vi "preparePubDataSVs.vi"(8 "error in (no error)":errorcluster, 11 "Model in":refnum<class "Model.lvclass">) -> (0 "error out":errorcluster, 3 "Model out":refnum<class "Model.lvclass">)   [LabVIEW 2015, in "Model.lvclass"]
doc: "Opens references to the PubDataSVs.\nDetermines the URLs from the configuration and the array of PubDataSVs.\nUpdate the array of PubDataSVs for each component."
uses:
  Model.lvclass
  ComponentTemplateCore/ComponentModel/ComponentModel/Typedefs/CommunicationConfig.ctl
  Typedefs/PubDataSV.ctl
  ComponentTemplateCore/ComponentModel/ComponentModel/Typedefs/SVProcessConfig.ctl
  Model.lvclass/Model.ctl
  Target/Target/Target.lvclass
  Typedefs/EXATypedefs.lvlib
  <vilib>/Utility/VariantDataType/VariantType.lvlib
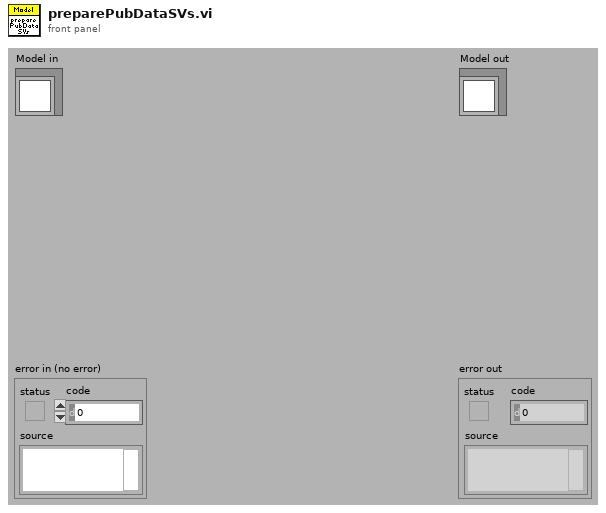
[diagram p1: front panel]
types:
  T1 = typedef "SVProcessConfig.ctl" = cluster{"subDataProcessPrototype":string, "pubDataProcessPrototype":string, "commandProcessPrototype":string, "commandSVName":string}
  T2 = typedef "EXATypedefs.lvlib/PubDataSV.ctl" = enum16{"DetailedState", "ErrorCode", "Heartbeat", "LoopTime_ms", "LoopTimeOutOfRange", "SummaryState", "Timestamp"}
  T3 = typedef "CommunicationConfig.ctl" = cluster{"hostComputerAddress":string, "ComponentAcronym":string, "InstanceIdentifier":i32}
  T4 = cluster{"Read Access":enum8{"Allowed", "Required", "None"}, "Write Access":enum8{"Allowed", "Required", "None"}}
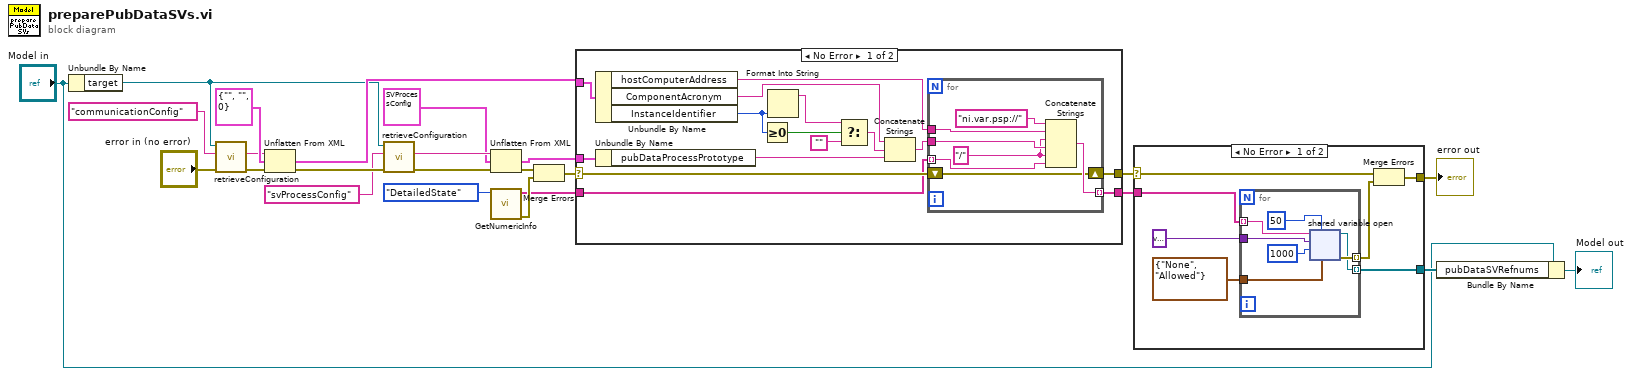
[diagram p0: block diagram]
diagram:
  n1 = Unbundle By Name("Model in") -> ("target"=w1:refnum<class "Target.lvclass">)
  n2 = call-dynamic "retrieveConfiguration.vi"("error in (no error)"="error in (no error)", "dataName"="communicationConfig", "Target in"=w1) -> ("error out"=w15:errorcluster, "dataValueFromFile"=w17:string)  [unwired: 6 in, 1 out]
  n3 = Unflatten From XML(xml string=w17, type=T3 {"hostComputerAddress"="", "ComponentAcronym"="", "InstanceIdentifier"=0} ("sharedVariableLibrariesConfig"), error in (no error)=w15) -> (value=w7:T3, error out=w6:errorcluster)
  n4 = call-dynamic "retrieveConfiguration.vi"("error in (no error)"=w6, "dataName"="svProcessConfig", "Target in"=w1) -> ("error out"=w5:errorcluster, "dataValueFromFile"=w9:string)  [unwired: 6 in, 1 out]
  n5 = Unflatten From XML(xml string=w9, type=T1 {"subDataProcessPrototype"="SubDataSV", "pubDataProcessPrototype"="PubDataSV", "commandProcessPrototype"="CommandSV", "commandSVName"="Command"} ("svProcessConfig"), error in (no error)=w5) -> (value=w2:T1, error out=w4:errorcluster)
  n6 = call <vilib>:"GetNumericInfo.vi"("Variant"=PubDataSV."DetailedState" ("PubDataSV")) -> ("error out"=w13:errorcluster, "EnumNames"=w11:string[])  [unwired: 7 in, 2 out]
  n7 = Merge Errors(w4, w13) -> (w12:errorcluster)
  n8 = case shown="No Error" w12 {
    selector: w12 -> [w34 w47]
    tunnel: [w39 _] -> w21
    tunnel: w7 -> [w37 _]
    tunnel: [w33 w47] -> w22
    tunnel: w11 -> [w27 _]
    tunnel: w2 -> [w26 _]
    frame No Error {
      n9 = Unbundle By Name(w37) -> ("hostComputerAddress"=w36:string, "ComponentAcronym"=w38:string, "InstanceIdentifier"=w32:i32)
      n10 = Unbundle By Name(w26) -> ("pubDataProcessPrototype"=w25:string)
      n11 = Greater Or Equal To 0?(x=w32) -> (x >= 0?=w31:bool)
      n12 = Format Into String(w32) -> (resulting string=w30:string)  [unwired: 3 in, 1 out]
      n13 = Select(t=w30, s=w31, f="") -> (s? t:f=w28:string)
      n14 = Concatenate Strings(w38, w28, w25) -> (w35:string)
      n15 = for {
        tunnel: w36 -> [w45]
        tunnel: w35 -> [w44]
        tunnel: [w42] -> w39 mode=indexing
        shift-right: [w40] -> w33
        shift-left: w34 -> [w40]
        tunnel: w27 -> [w41] mode=indexing
        w43 = "/" ("string")
        n16 = Concatenate Strings("ni.var.psp://" ("string"), w45, w43, w44, w43, w41) -> (w42:string)
      }
    }
    frame Error {
    }
  }
  n17 = case shown="No Error" w22 {
    selector: w22 -> [w52 w62]
    tunnel: w21 -> [w53 _]
    tunnel: [w49 w62] -> w20
    tunnel: [w48 _] -> w19
    frame No Error {
      n18 = for {
        tunnel: T4 {"Read Access"=enum."None", "Write Access"=enum."Allowed"} ("access") -> [w61]
        tunnel: w53 -> [w60] mode=indexing
        tunnel: [w58] -> w48 mode=indexing
        tunnel: variant ("variant") -> [w57]
        tunnel: [w59] -> w51 mode=indexing
        n19 = shared-variable-open(w60, w57, w61, 1000 ("timeout ms"), u32 50 ("buffer size in elements")) -> (w58:refnum<k21>, w59:errorcluster)  [unwired: 1 in]
      }
      n20 = Merge Errors(w52, w51) -> (w49:errorcluster)
    }
    frame Error {
    }
  }
  "error out" <- w20
  n21 = Bundle By Name(cluster="Model in", "pubDataSVRefnums"=w19) -> (→"Model out":refnum<class "Model.lvclass">)
